vi "Volume Demo.vi"() -> ()   [LabVIEW 2012]
uses:
  LabVIEW/user.lib/SpectralRadar.llb/set Scan Output.vi
  LabVIEW/user.lib/SpectralRadar.llb/set Spectrum Output.vi
  LabVIEW/user.lib/SpectralRadar.llb/display Data 2D.vi
  LabVIEW/user.lib/SpectralRadar.llb/OCT Device.lvclass
  LabVIEW/user.lib/SpectralRadar.llb/Probe.lvclass
  LabVIEW/user.lib/SpectralRadar.llb/Processing.lvclass
  LabVIEW/user.lib/SpectralRadar.llb/Scan Pattern.lvclass
  LabVIEW/user.lib/SpectralRadar.llb/Data.lvclass
  LabVIEW/user.lib/SpectralRadar.llb/Raw Data.lvclass
panel:
  in  "BScans / Volume":i32=256
  in  "AScans / BScan":i32=256
  in  "Range Y [mm]":dbl=1.0
  in  "Range X [mm]":dbl=1.0
  out "Spectral Data":dbl[][](graph)
  out "B-Scan Data":dbl[][](graph)
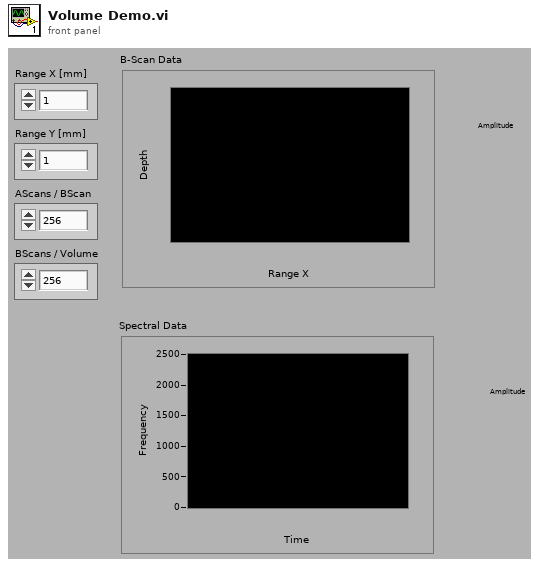
[diagram p1: front panel]
types:
  T1 = enum16{"Asynchronous Continuous", "Asynchronous Finite", "Synchronous"}
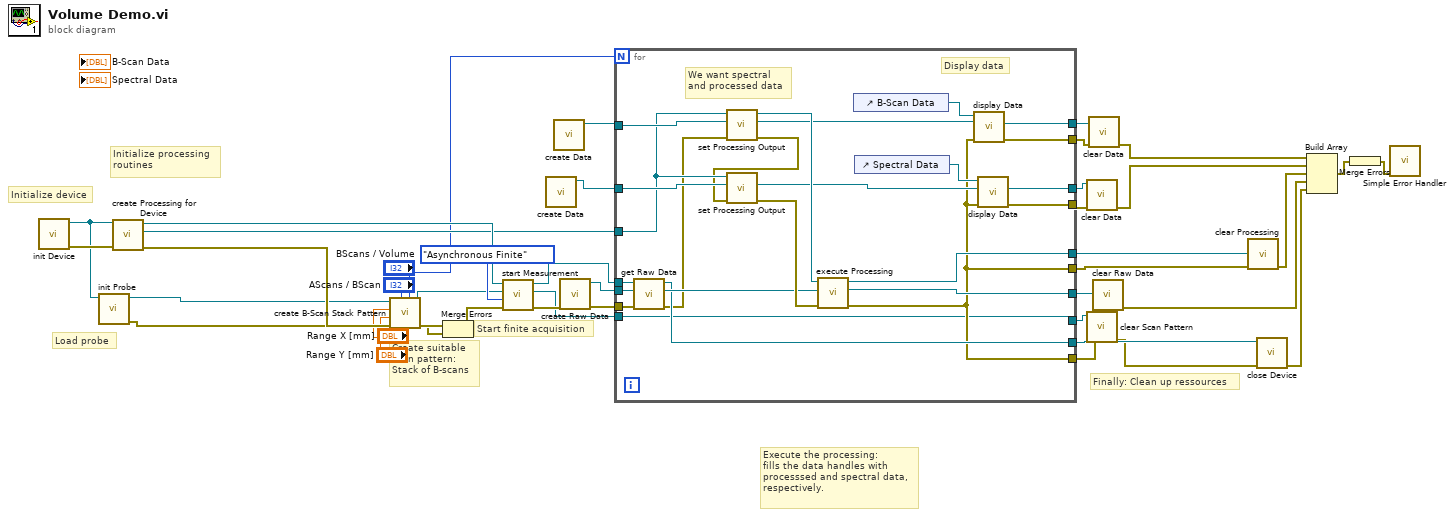
[diagram p0: block diagram]
diagram:
  # "Finally: Clean up ressources"
  # "Start finite acquisition"
  # "Create suitable\nscan pattern:\nStack of B-scans"
  # "Execute the processing:\nfills the data handles with \nprocesssed and spectral data,\nrespectively."
  # "Load probe"
  # "Initialize processing \nroutines"
  # "Initialize device"
  n1 = call "init Device.vi"() -> ("error out"=w40:errorcluster, "OCTDevice"=w26:refnum<class "OCT Device.lvclass">)  [unwired: 6 in]
  n2 = call "init Probe.vi"("OCT Device"=w26) -> ("error out"=w32:errorcluster, "GalvoControl"=w33:refnum<class "Probe.lvclass">)  [unwired: 5 in]
  n3 = call "create Processing for Device.vi"("error in (no error)"=w40, "OCTDevice"=w26) -> ("error out"=w39:errorcluster, "Processing"=w37:refnum<class "Processing.lvclass">, "OCTDevice"=w38:refnum<class "OCT Device.lvclass">)  [unwired: 3 in]
  n4 = call "create B-Scan Stack Pattern.vi"("Size Y"="BScans / Volume", "Size X"="AScans / BScan", "error in (no error)"=w32, "Range Y"="Range Y [mm]", "Range X"="Range X [mm]", "Probe"=w33) -> ("error out"=w15:errorcluster, "Scan Pattern"=w13:refnum<class "Scan Pattern.lvclass">)  [unwired: 1 in, 1 out]
  n5 = Merge Errors(w39, w15) -> (w23:errorcluster)
  n6 = call "start Measurement.vi"("error in (no error)"=w23, "Acquisition Type"=T1."Asynchronous Finite", "Scan Pattern"=w13, "OCTDevice"=w38) -> ("error out"=w21:errorcluster, "Scan Pattern"=w11:refnum<class "Scan Pattern.lvclass">, "OCTDevice"=w12:refnum<class "OCT Device.lvclass">)  [unwired: 1 in]
  n7 = call "create Data.vi"() -> ("Data"=w7:refnum<class "Data.lvclass">)  [unwired: 6 in, 1 out]
  n8 = call "create Data.vi"() -> ("Data"=w8:refnum<class "Data.lvclass">)  [unwired: 6 in, 1 out]
  n9 = call "create Raw Data.vi"("error in (no error)"=w21) -> ("error out"=w20:errorcluster, "Raw Data"=w22:refnum<class "Raw Data.lvclass">)  [unwired: 5 in]
  n10 = for {
    N: "BScans / Volume" -> [_]
    tunnel: w22 -> [w63]
    tunnel: w12 -> [w64]
    tunnel: w20 -> [w62]
    tunnel: w37 -> [w59]
    tunnel: w7 -> [w61]
    tunnel: w8 -> [w60]
    tunnel: [w50] -> w19
    tunnel: [w49] -> w35
    tunnel: [w48] -> w3
    tunnel: [w47] -> w6
    tunnel: [w46] -> w2
    tunnel: [w45] -> w5
    tunnel: [w44] -> w36
    tunnel: [w42] -> w34
    tunnel: [w42] -> w9
    tunnel: [w41] -> w10
    tunnel: w11 -> [w41]
    # "Display data"
    # "We want spectral\nand processed data"
    n11 = call "get Raw Data.vi"("error in (no error)"=w62, "RawData in"=w63, "OCTDevice in"=w64) -> ("error out"=w43:errorcluster, "RawData out"=w55:refnum<class "Raw Data.lvclass">, "OCTDevice out"=w44:refnum<class "OCT Device.lvclass">)  [unwired: 2 in]
    n12 = call-poly "set Processing Output.vi"("error in (no error)"=w43, "Data"=w60, "Processing"=w59) -> ("error out"=w57:errorcluster, "Data"=w53:refnum<class "Data.lvclass">, "Processing"=w58:refnum<class "Processing.lvclass">)  [unwired: 2 in]
    n13 = call-poly "set Processing Output.vi"("error in (no error)"=w57, "Data"=w61, "Processing"=w59) -> ("error out"=w56:errorcluster, "Data"=w51:refnum<class "Data.lvclass">)  [unwired: 2 in, 1 out]
    n14 = call "execute Processing.vi"("error in (no error)"=w56, "Raw Data"=w55, "Processing"=w58) -> ("error out"=w42:errorcluster, "Raw Data"=w50:refnum<class "Raw Data.lvclass">, "Processing"=w49:refnum<class "Processing.lvclass">)  [unwired: 2 in]
    n15 = control-ref of="B-Scan Data"() -> (w54:refnum<vi>)
    n16 = control-ref of="Spectral Data"() -> (w52:refnum<vi>)
    n17 = call-poly "display Data.vi"("error in (no error)"=w42, "Data in"=w53, "IntGraph Refnum"=w54) -> ("error out"=w45:errorcluster, "Data out"=w47:refnum<class "Data.lvclass">)  [unwired: 2 in, 1 out]
    n18 = call-poly "display Data.vi"("error in (no error)"=w42, "Data in"=w51, "IntGraph Refnum"=w52) -> ("error out"=w46:errorcluster, "Data out"=w48:refnum<class "Data.lvclass">)  [unwired: 2 in, 1 out]
  }
  n19 = call "clear Data.vi"("error in (no error)"=w2, "Data"=w3) -> ("error out"=w1:errorcluster)  [unwired: 5 in]
  n20 = call "clear Scan Pattern.vi"("error in (no error)"=w9, "Scan Pattern in"=w10) -> ("error out"=w25:errorcluster)  [unwired: 5 in]
  n21 = call "clear Data.vi"("error in (no error)"=w5, "Data"=w6) -> ("error out"=w4:errorcluster)  [unwired: 5 in]
  n22 = call "clear Raw Data.vi"("Raw Data"=w19) -> ("error out"=w30:errorcluster)  [unwired: 6 in]
  n23 = call "clear Processing.vi"("error in (no error)"=w34, "Processing"=w35) -> ("error out"=w31:errorcluster)  [unwired: 5 in]
  n24 = call "close Device.vi"("error in (no error)"=w25, "OCTDevice"=w36) -> ("error out"=w29:errorcluster)  [unwired: 5 in]
  n25 = Build Array(w4, w1, w31, w30, w29) -> (w28:errorcluster[])
  n26 = Merge Errors(w28) -> (w27:errorcluster)
  n27 = call <vilib>:"Simple Error Handler.vi"("error in (no error)"=w27) -> ()  [unwired: 4 in, 5 out]
